vi "SelectMethodsOfInterfaces.vi"(8 "error in":errorcluster, 11 "InterfacePath":T1[](array[typedef])=[{"Name(Short if no Conflicts)"="Sub_Interface1", "FullQualifierName"="Sub_Interface1.lvclass", "Description"="", "Path"=path "C:/Projects/Interface/Sub_Interface1/Sub_Interface1.lvclass", "ParentInterfaceNames(Short if no Conflitcs)"=[], "ParentInterfaceFullQualifierNames"=[], "IconPath"=path "C:/Program Files (x86)/National Instruments/LabVIEW 2020/resource/Framework/Providers/Open_GDS/icons/InterfaceBlue.png", "Methods"=[{"Name"="Add.vi", "Descriptions"="This is an Add Interface Method", "RelativePath"=path "../Add.vi", "SourceScope"=enum."public", "MustOverride"=TRUE, "VirtualFolderLocation"=["Folder"]}, {"Name"="Execute.vi", "Descriptions"="", "RelativePath"=path "../Execute.vi", "SourceScope"=enum."public", "MustOverride"=TRUE, "VirtualFolderLocation"=[]}]}, {"Name(Short if no Conflicts)"="Interface1", "FullQualifierName"="Interface1.lvclass", "Description"="", "Path"=path "C:/Projects/Interface/Interface1/Interface1.lvclass", "ParentInterfaceNames(Short if no Conflitcs)"=["Sub_Interface1"], "ParentInterfaceFullQualifierNames"=["Sub_Interface1.lvclass"], "IconPath"=path "C:/Program Files (x86)/National Instruments/LabVIEW 2020/resource/Framework/Providers/Open_GDS/icons/InterfaceBrown.png", "Methods"=[{"Name"="Execute2.vi", "Descriptions"="", "RelativePath"=path "../Execute2.vi", "SourceScope"=enum."public", "MustOverride"=TRUE, "VirtualFolderLocation"=[]}, {"Name"="", "Descriptions"="", "RelativePath"=path "", "SourceScope"=enum."invalid scope", "MustOverride"=FALSE, "VirtualFolderLocation"=[]}]}]) -> (0 "error out":errorcluster, 3 "MethodsPerInterface(Empty=>All)":cluster{"Methods":string[]}[](array[cluster]))   [LabVIEW 2020, in "InterfaceLibrary.lvlib"]
uses:
  <resource>/Framework/Providers/Open_GDS/ClassProviders/Common/InterfaceLibrary/InterfaceLibrary.lvlib
  <resource>/Framework/Providers/Open_GDS/ClassProviders/Common/LvClass_class/GDSLvClass_ClassMethodInfo.ctl
  <resource>/Framework/Providers/Open_GDS/ClassProviders/Common/InterfaceLibrary/InterfaceInfo.ctl
panel:
  in  "Tree":string(tree) caption="No methods selected"
  in  "Cancel":bool
  in  "Ok":bool
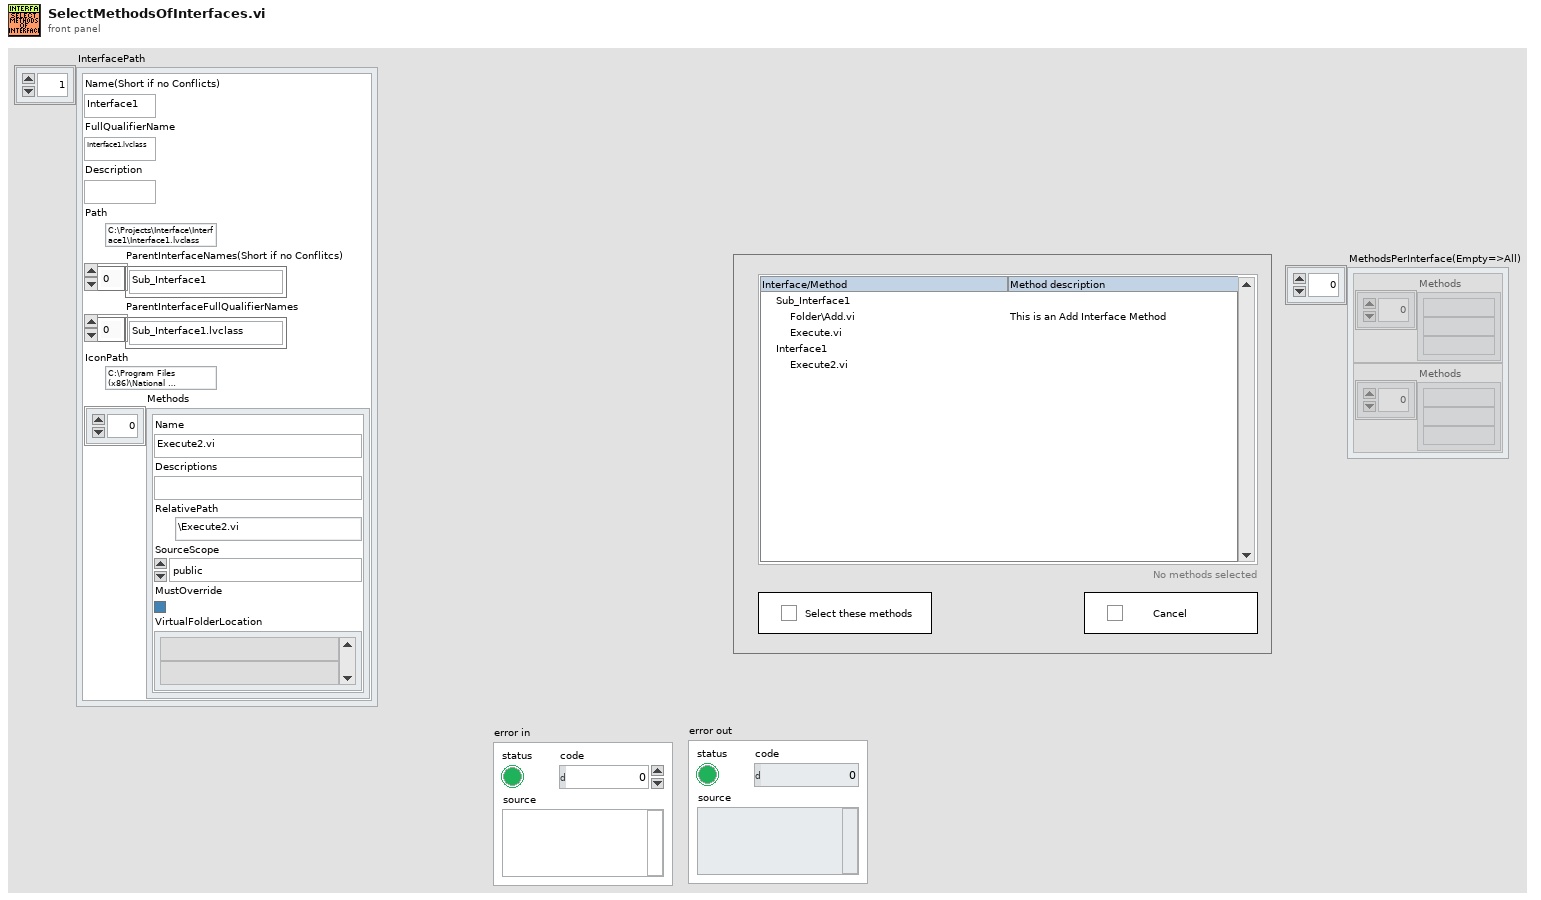
[diagram p1: front panel]
types:
  T1 = typedef "InterfaceLibrary.lvlib/InterfaceInfo.ctl" = cluster{"Name(Short if no Conflicts)":string, "FullQualifierName":string, "Description":string, "Path":path, "ParentInterfaceNames(Short if no Conflitcs)":string[], "ParentInterfaceFullQualifierNames":string[], "IconPath":path, "Methods":T2[]}
  T2 = typedef "GDSLvClass_ClassMethodInfo.ctl" = cluster{"Name":string, "Descriptions":string, "RelativePath":path, "SourceScope":enum32{"invalid scope", "public", "private", "protected", "community"}, "MustOverride":bool, "VirtualFolderLocation":string[]}
  T3 = typedef "LVPoint32TypeDef.ctl" = cluster{"Horizontal":i32, "Vertical":i32}
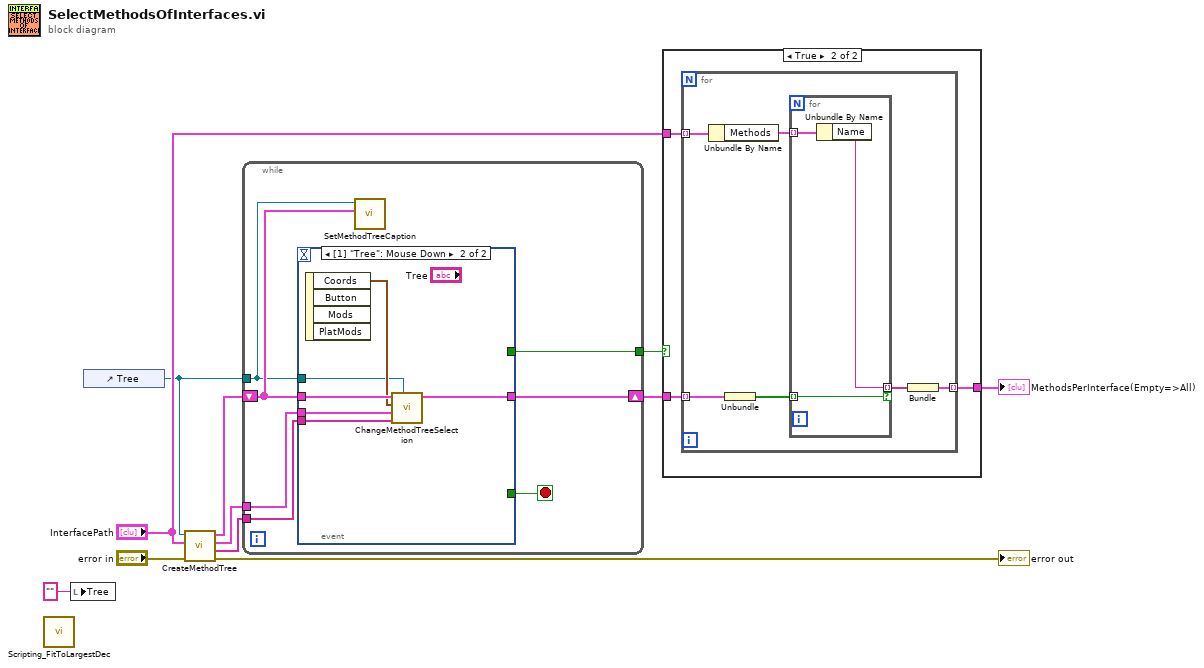
[diagram p0: block diagram]
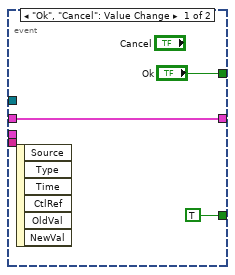
[diagram p2: hidden frame]
diagram:
  n1 = call <resource>:"Scripting_FitToLargestDec.vi"() -> ()  [unwired: 6 in, 2 out]
  n2 = local write "Tree"("" ("Tree")) -> ()
  n3 = control-ref of="Tree"() -> (w1:refnum<vi>)
  n4 = call <resource>:"CreateMethodTree.vi"("error in (no error)"="error in", "InterfacePath"="InterfacePath", "TreeControlRef"=w1) -> ("error out"=→"error out":errorcluster, "InterfacesTag"=w9:string[], "MethodsTagPerInterfaces"=w8:cluster{"Array":string[]}[], "MethodsSelectedPerInterface"=w7:cluster{"Array":bool[]}[])  [unwired: 4 in, 1 out]
  n5 = while {
    tunnel: w9 -> [w17]
    tunnel: w8 -> [w16]
    shift-right: [w14] -> w5
    shift-left: w7 -> [w15]
    tunnel: [w13] -> w6
    tunnel: w1 -> [w12]
    stop <- w18 stop-if-true
    n6 = event shown="[1] \"Tree\": Mouse Down" {
      selector: _ -> [_ _]
      dyn-events: _ -> [_ _]
      timeout: _ -> [_ _]
      tunnel: [TRUE _] -> w18
      tunnel: w17 -> [_ w23]
      tunnel: w16 -> [_ w27]
      tunnel: w15 -> [w20 w25]
      tunnel: [w20 w26] -> w14
      tunnel: ["Ok" _] -> w13
      tunnel: w12 -> [_ w22]
      event "Ok", "Cancel": Value Change {
        n7 = event-data() -> ()  [unwired: 1 in, 6 out]
      }
      event "Tree": Mouse Down {
        n8 = event-data() -> ("Coords"=w24:T3)  [unwired: 1 in, 3 out]
        n9 = call <resource>:"ChangeMethodTreeSelection.vi"("TreeControl in"=w22, "Interfaces"=w23, "MethodsPerInterfaces"=w27, "MouseClickCoordinates"=w24, "SelectedMethodsIn"=w25) -> ("SelectedMethodsOut"=w26:cluster{"Array":bool[]}[])  [unwired: 6 in]
      }
    }
    n10 = call <resource>:"SetMethodTreeCaption.vi"("MethodsSelectedPerInt"=w15, "TreeControl in"=w12) -> ()  [unwired: 9 in, 1 out]
  }
  n11 = case shown="True" w6 {
    tunnel: w5 -> [_ w30]
    tunnel: "InterfacePath" -> [_ w29]
    tunnel: [_ w28] -> w3
    frame False {
    }
    frame True {
      n12 = for {
        tunnel: w30 -> [w36] mode=indexing
        tunnel: w29 -> [w35] mode=indexing
        tunnel: [w31] -> w28 mode=indexing
        n13 = Unbundle By Name(w35) -> ("Methods"=w34:T2[])
        n14 = Unbundle(w36) -> ("Array"=w33:bool[])
        n15 = for {
          tunnel: w34 -> [w39] mode=indexing
          tunnel: w33 -> [w37] mode=indexing
          tunnel: [w38] -> w32 mode=indexing if=w37
          n16 = Unbundle By Name(w39) -> ("Name"=w38:string)
        }
        n17 = Bundle(w32) -> (w31:cluster{string[]})  [unwired: 1 in]
      }
    }
  }
  "MethodsPerInterface(Empty=>All)" <- w3
